vi "ex_ExcelAllConfig.vi"(11 "timestamp input":T1={"absolute time"=FALSE, "Timestamp format"="hh:mm:ss.000"} caption="timestamp") -> (2 "Cancel?":bool, 3 "timestamp output":T1={"absolute time"=FALSE, "Timestamp format"="hh:mm:ss.000"} caption="timestamp")   [LabVIEW 2017]
uses:
  <vilib>/express/express output/ExFileWriteBlock.llb/ex_ExcelAdvancedConfig.ctl
panel:
  in  "Format":string
  in  "Absolute":bool=TRUE
  in  "Cancel":bool
  in  "OK":bool
  in  "Help":bool
  # "Timestamp"
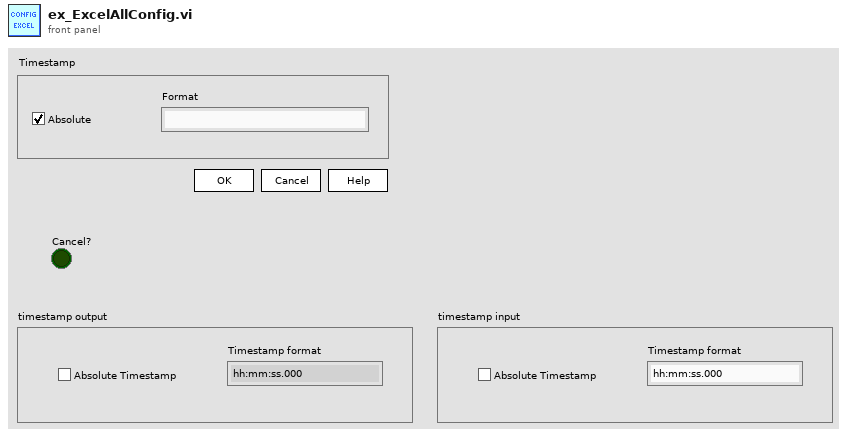
[diagram p1: front panel]
types:
  T1 = typedef "ex_ExcelAdvancedConfig.ctl" = cluster{"absolute time":bool, "Timestamp format":string}
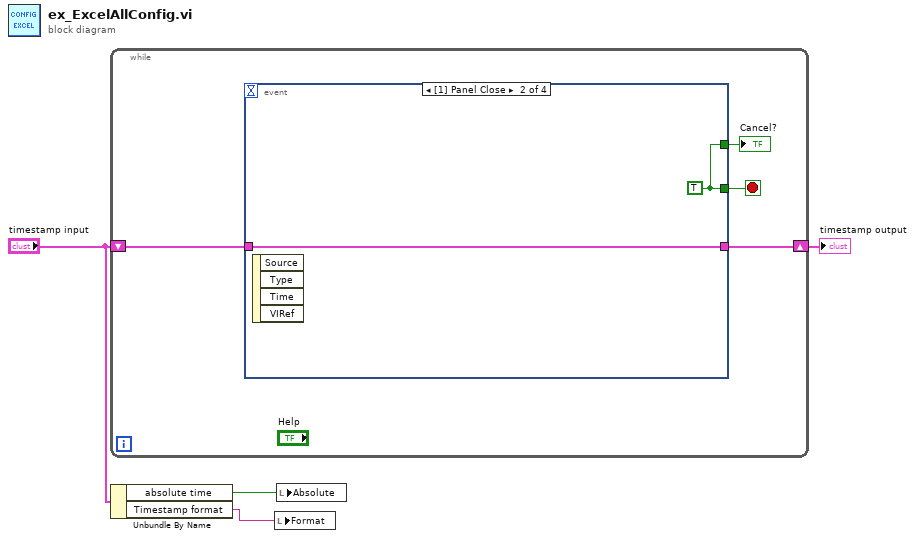
[diagram p0: block diagram]
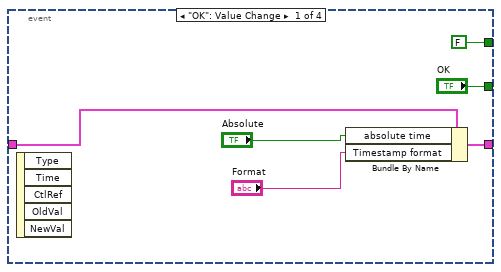
[diagram p2: hidden frame]
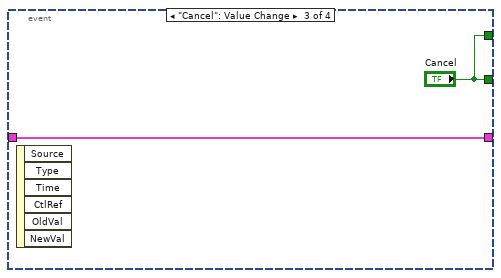
[diagram p3: hidden frame]
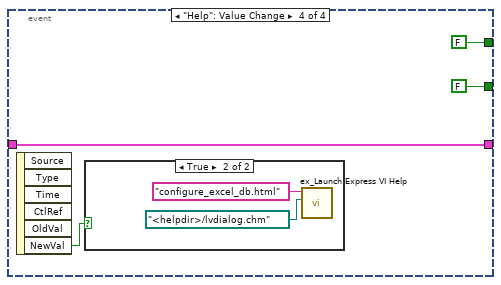
[diagram p4: hidden frame]
diagram:
  n1 = while {
    shift-right: [w6] -> w4
    shift-left: "timestamp input" -> [w7]
    stop <- w8 stop-if-true
    n2 = event shown="[1] Panel Close" {
      selector: _ -> [_ _ _ _]
      dyn-events: _ -> [_ _ _ _]
      timeout: _ -> [_ _ _ _]
      tunnel: ["OK" w15 "Cancel" FALSE ("Cancel")] -> w8
      tunnel: [w12 w16 w18 w20] -> w6
      tunnel: w7 -> [w13 w16 w18 w20]
      tunnel: [FALSE ("Cancel") w15 "Cancel" FALSE ("Cancel")] -> w5
      event "OK": Value Change {
        n3 = event-data() -> ()  [unwired: 6 out]
        n4 = Bundle By Name(cluster=w13, "absolute time"="Absolute", "Timestamp format"="Format") -> (w12:T1)
      }
      event Panel Close {
        w15 = TRUE
        n5 = event-data() -> ()  [unwired: 5 out]
      }
      event "Cancel": Value Change {
        n6 = event-data() -> ()  [unwired: 7 out]
      }
      event "Help": Value Change {
        n7 = event-data() -> ("NewVal"=w22:bool)  [unwired: 6 out]
        n8 = case shown="True" w22 {
          frame False {
          }
          frame True {
            n9 = call <vilib>:"ex_Launch Express VI Help.vi"("Help File Path"=path "<helpdir>/lvdialog.chm", "Keyword/HTML File"="configure_excel_db.html") -> ()  [unwired: 1 in, 5 out]
          }
        }
      }
    }
    "Cancel?" <- w5
  }
  "timestamp output" <- w4
  n10 = Unbundle By Name("timestamp input") -> ("absolute time"=w2:bool, "Timestamp format"=w1:string)
  n11 = local write "Format"(w1) -> ()
  n12 = local write "Absolute"(w2) -> ()
